vi "Periodic Tasks.vi"() -> ()   [LabVIEW 2011]
doc: "This VI runs in parallel to other tasks. It can contain as many user-defined periodic loops as you need. These can carry out PID or other sorts of timed response."
uses:
  <vilib>/Rock Robotics/SystemInterfaces/Utilities/FPGA_UtilitiesLED State.ctl
  <vilib>/Rock Robotics/SystemInterfaces/Utilities/FPGA_UtilitiesLED Source.ctl
  <vilib>/Rock Robotics/WPI/Relay/WPI_RelayValue.ctl
  Robot Global Data.vi
panel:
  out "Rate":dbl
  out "Heading 2":u16
  out "Angular Rate":dbl
  out "Angle":dbl
  out "Direction":bool
  out "Distance":dbl
  in  "Home Speed":dbl=1.0
  in  "Home Position":dbl=2.85
  out "Current Voltage":dbl
  in  "upper limit":dbl=4.5
  in  "lower limit":dbl=0.85
  # "Speed to move to home"
  # "Target Tracking"
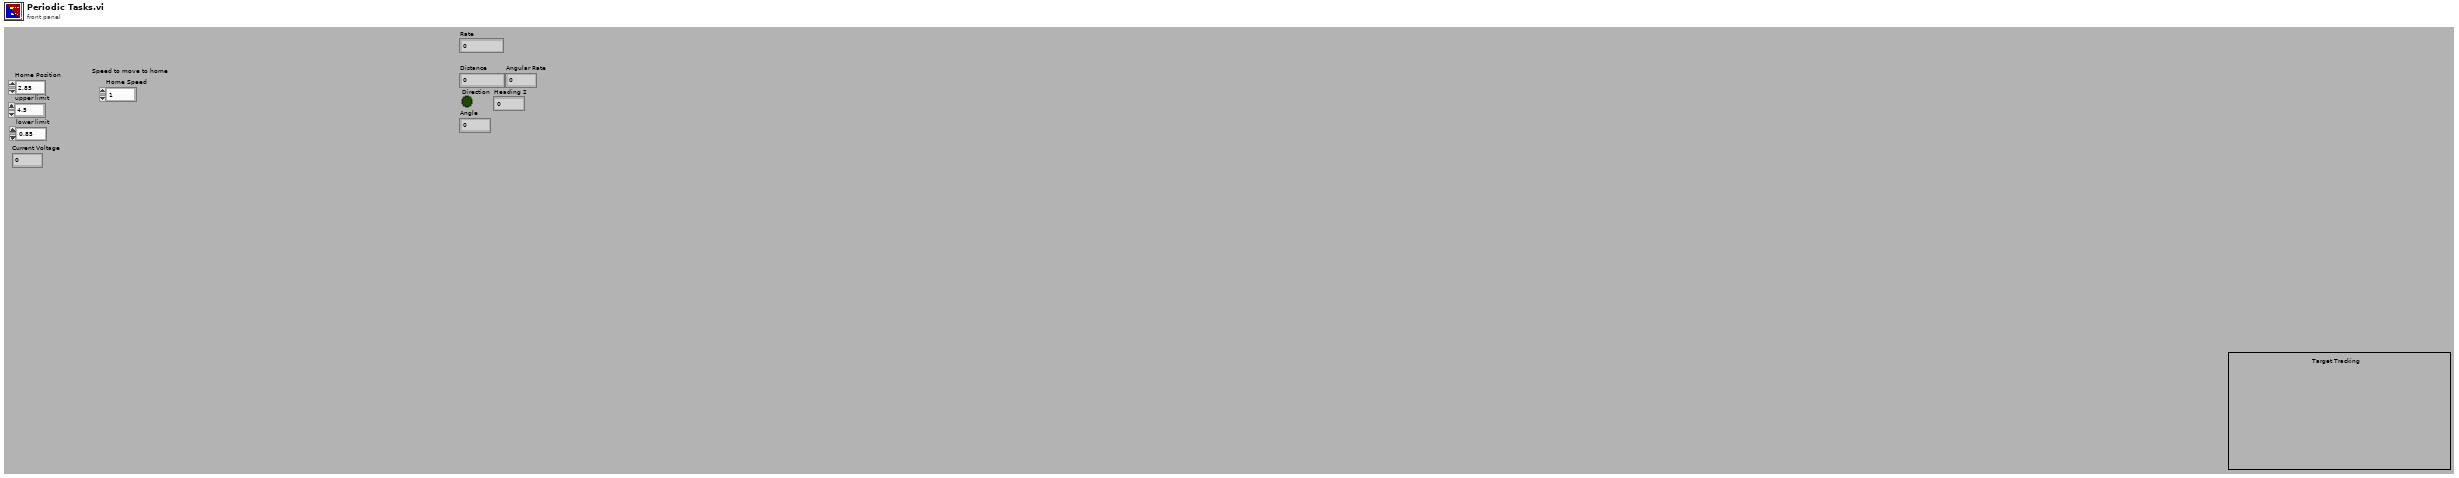
[diagram p1: front panel]
types:
  T1 = typedef "WPI_RelayValue.ctl" = enum16{"Off", "On", "Forward", "Reverse"}
  T2 = typedef "WPI_GyroDevRef.ctl" = cluster{"DevStatus":errorcluster, "Analog Module":T3, "Analog Channel":T4, "Offset":dbl, "Gain (VoltsPerDegree/Second)":dbl}
  T3 = typedef "FPGA_TypedefAnalogModule.ctl" = enum16{"Analog Module 1", "Analog Module 2"}
  T4 = typedef "FPGA_AIChannel.ctl" = enum8{"AI 1", "AI 2", "AI 3", "AI 4", "AI 5", "AI 6", "AI 7", "AI 8", "Invalid"}
  T5 = typedef "WPI_EncoderDevRef.ctl" = cluster{"DevStatus":errorcluster, "EncoderIndex":T6, "CounterIndex":T7, "DistancePerCount":dbl, "Decoding Type":T8}
  T6 = typedef "FPGA_EncoderIdx.ctl" = enum8{"Enc 0", "Enc 1", "Enc 2", "Enc 3", "Invalid"}
  T7 = typedef "FPGA_CounterCtrSystemIndex.ctl" = enum8{"Ctr 0", "Ctr 1", "Ctr 2", "Ctr 3", "Ctr 4", "Ctr 5", "Ctr 6", "Ctr 7", "Invalid"}
  T8 = typedef "WPI_EncoderType.ctl" = enum16{"1x", "2x", "4x"}
  T9 = typedef "WPI_AnalogChannelDevRef.ctl" = cluster{"DevStatus":errorcluster, "Analog Module":T3, "Analog Channel":T4}
  T10 = typedef "WPI_I2CDevRef.ctl" = cluster{"DevStatus":errorcluster, "Digital Module":T11, "Device Address":u8}
  T11 = typedef "FPGA_TypedefDigitalModule.ctl" = enum16{"Digital Module 1", "Digital Module 2"}
  T12 = typedef "WPI_RelayDevRef.ctl" = cluster{"DevStatus":errorcluster, "Relay Channel":T13, "Digital Module":T11, "Relay Direction":T14}
  T13 = typedef "FPGA_DIORelayChannel.ctl" = enum8{"Relay 1", "Relay 2", "Relay 3", "Relay 4", "Relay 5", "Relay 6", "Relay 7", "Relay 8", "Invalid"}
  T14 = typedef "WPI_RelayDirection.ctl" = enum16{"Both directions", "Forward only", "Reverse only"}
  T15 = cluster{"Driver Station Digital Output (1-8)[0]":bool, "Driver Station Digital Output (1-8)[1]":bool, "Driver Station Digital Output (1-8)[2]":bool, "Driver Station Digital Output (1-8)[3]":bool, "Driver Station Digital Output (1-8)[4]":bool, "Driver Station Digital Output (1-8)[5]":bool, "Driver Station Digital Output (1-8)[6]":bool, "Driver Station Digital Output (1-8)[7]":bool, "Driver Station Digital Output (1-8)[8]":bool}
  T16 = typedef "FPGA_UtilitiesLED State.ctl" = enum16{"Off", "On", "Toggle"}
  T17 = typedef "FPGA_UtilitiesLED Source.ctl" = enum16{"User LED", "FPGA LED"}
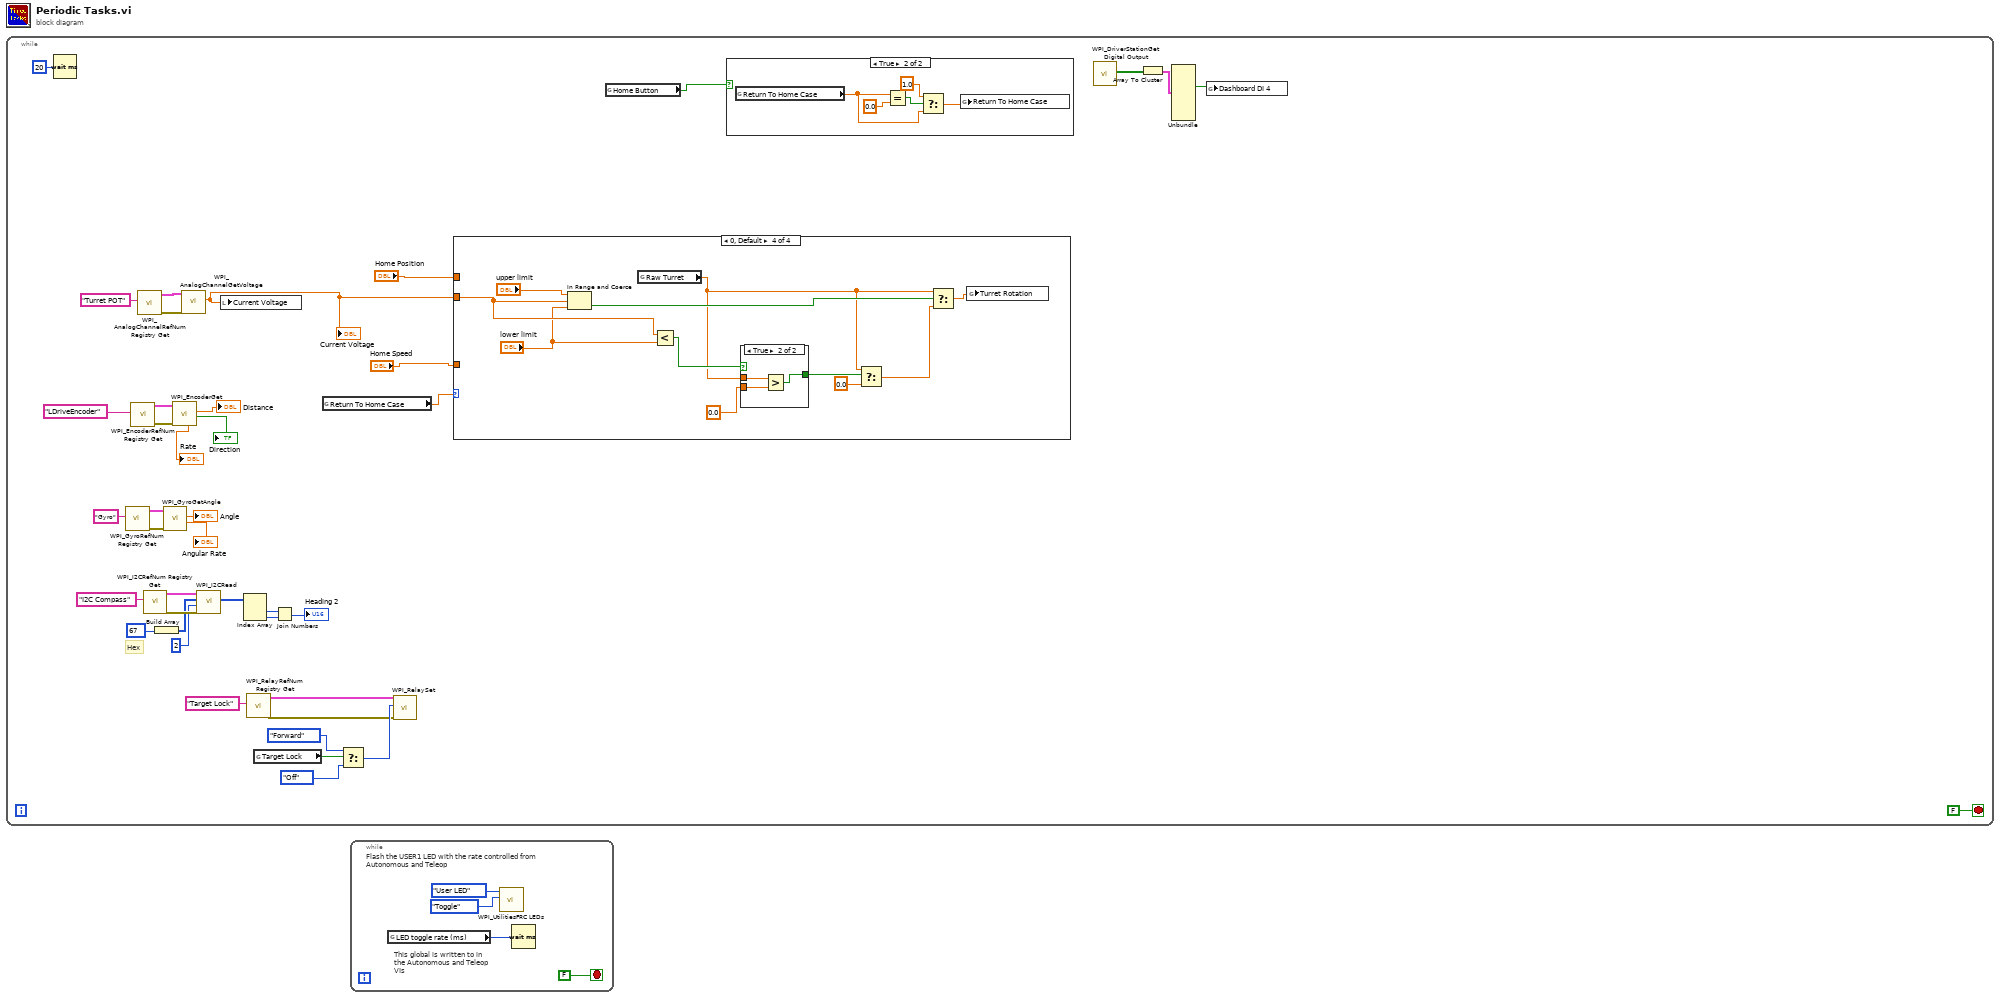
[diagram p0: block diagram]
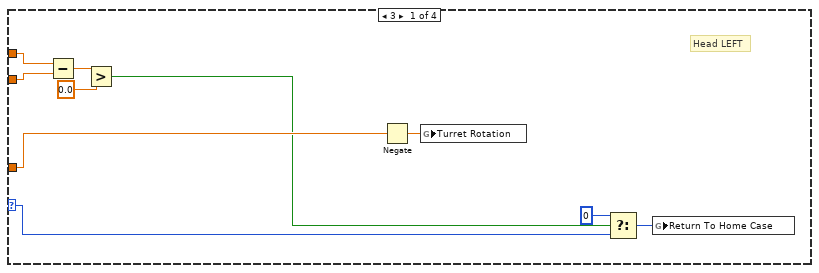
[diagram p2: hidden frame]
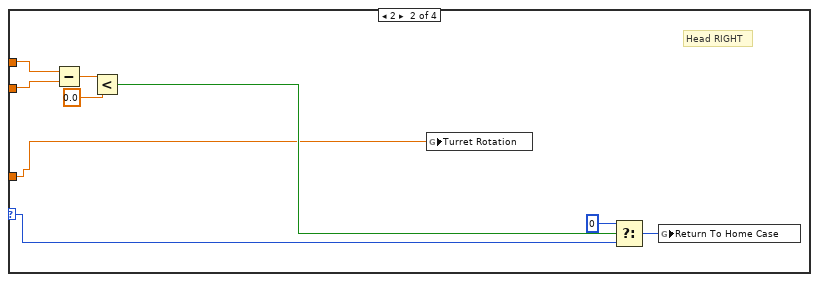
[diagram p3: hidden frame]
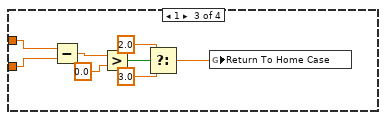
[diagram p4: hidden frame]
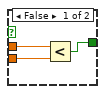
[diagram p5: hidden frame]
diagram:
  n1 = while {
    stop <- FALSE stop-if-true
    # "Hex"
    n2 = Wait (ms)(milliseconds to wait=u32 20) -> ()  [unwired: 1 out]
    n3 = call <vilib>:"WPI_GyroRefNum Registry Get.vi"("refnum name"="Gyro") -> ("error out"=w14:errorcluster, "GyroDevRef"=w15:T2)  [unwired: 9 in]
    n4 = call <vilib>:"WPI_EncoderRefNum Registry Get.vi"("refnum name"="LDriveEncoder") -> ("error out"=w18:errorcluster, "EncoderDevRef"=w19:T5)  [unwired: 9 in]
    n5 = call <vilib>:"WPI_AnalogChannelRefNum Registry Get.vi"("refnum name"="Turret POT") -> ("error out"=w21:errorcluster, "AIDeviceRef"=w22:T9)  [unwired: 9 in]
    n6 = call <vilib>:"WPI_I2CRefNum Registry Get.vi"("refnum name"="I2C Compass") -> ("error out"=w10:errorcluster, "I2CDevRef"=w9:T10)  [unwired: 9 in]
    n7 = Build Array(67) -> (w1:i32[])
    n8 = call <vilib>:"WPI_GyroGetAngle.vi"("error in (no error)"=w14, "GyroDevRef"=w15) -> ("Angular Rate"=→"Angular Rate":dbl, "Angle"=→"Angle":dbl)  [unwired: 6 in, 2 out]
    n9 = call <vilib>:"WPI_EncoderGet.vi"("error in (no error)"=w18, "EncoderDevRef"=w19) -> ("Direction"=→"Direction":bool, "Distance"=→"Distance":dbl, "Rate"=→"Rate":dbl)  [unwired: 4 in, 3 out]
    n10 = call <vilib>:"WPI_AnalogChannelGetVoltage.vi"("error in (no error)"=w21, "AIDeviceRef"=w22) -> ("Voltage"=w30:dbl)  [unwired: 7 in, 2 out]
    "Current Voltage" <- w30
    n11 = call <vilib>:"WPI_I2CRead.vi"("error in (no error)"=w10, "I2CBytesToRead"=u8 2, "I2CRegister"=w1, "I2CDevRef"=w9) -> ("Data Out"=w7:u8[])  [unwired: 5 in, 2 out]
    n12 = local write "Current Voltage"(w30) -> ()
    n13 = Index Array(array=w7) -> (element #1=w5:u8, element #2=w6:u8)  [unwired: 2 in]
    n14 = call <vilib>:"WPI_RelayRefNum Registry Get.vi"("refnum name"="Target Lock") -> ("error out"=w32:errorcluster, "RelayDevRef"=w33:T12)  [unwired: 9 in]
    n15 = global read "Robot Global Data.vi" "Target Lock"() -> (w38:bool)
    n16 = Join Numbers(hi=w5, lo=w6) -> ((hi.lo)=→"Heading 2":u16)
    n17 = global read "Robot Global Data.vi" "Return To Home Case"() -> (w29:dbl)
    n18 = Select(t=WPI_RelayValue."Forward" ("RelayValue"), s=w38, f=WPI_RelayValue."Off" ("RelayValue")) -> (s? t:f=w35:T1)
    n19 = call <vilib>:"WPI_RelaySet.vi"("error in (no error)"=w32, "RelayValue"=w35, "RelayDevRef"=w33) -> ()  [unwired: 7 in, 2 out]
    n20 = case shown="0, Default" w29 {
      selector: w29 -> [w49 w53 _ _]
      tunnel: w30 -> [w45 w54 w67 w79]
      tunnel: "Home Position" -> [w46 w55 w68 _]
      tunnel: "Home Speed" -> [w47 w52 _ _]
      frame 3 {
        # "Head LEFT"
        n21 = Subtract(x=w46, y=w45) -> (x-y=w44:dbl)
        n22 = Greater?(x=w44, y=0.0) -> (0:w42:bool)
        n23 = Negate(x=w47) -> (-x=w48:dbl)
        n24 = global write "Robot Global Data.vi" "Turret Rotation"(w48) -> ()
        n25 = Select(t=0, s=w42, f=w49) -> (s? t:f=w50:i32)
        n26 = global write "Robot Global Data.vi" "Return To Home Case"(w50) -> ()
      }
      frame 2 {
        # "Head RIGHT"
        n27 = Subtract(x=w55, y=w54) -> (x-y=w58:dbl)
        n28 = Less?(x=w58, y=0.0) -> (x < y?=w56:bool)
        n29 = global write "Robot Global Data.vi" "Turret Rotation"(w52) -> ()
        n30 = Select(t=0, s=w56, f=w53) -> (s? t:f=w59:i32)
        n31 = global write "Robot Global Data.vi" "Return To Home Case"(w59) -> ()
      }
      frame 1 {
        n32 = Subtract(x=w68, y=w67) -> (x-y=w66:dbl)
        n33 = Greater?(x=w66, y=0.0) -> (0:w64:bool)
        n34 = Select(t=2.0, s=w64, f=3.0) -> (s? t:f=w61:dbl)
        n35 = global write "Robot Global Data.vi" "Return To Home Case"(w61) -> ()
      }
      frame 0, Default {
        n36 = In Range and Coerce(upper limit="upper limit", x=w79, lower limit="lower limit") -> (In Range?=w76:bool)  [unwired: 1 out]
        n37 = global read "Robot Global Data.vi" "Raw Turret"() -> (w69:dbl)
        n38 = Less?(x=w79, y="lower limit") -> (x < y?=w71:bool)
        n39 = case shown="True" w71 {
          tunnel: 0.0 -> [w81 w85]
          tunnel: [w80 w84] -> w72
          tunnel: w69 -> [w82 w83]
          frame False {
            n40 = Less?(x=w82, y=w81) -> (x < y?=w80:bool)
          }
          frame True {
            n41 = Greater?(x=w83, y=w85) -> (0:w84:bool)
          }
        }
        n42 = Select(t=w69, s=w72, f=0.0) -> (s? t:f=w70:dbl)
        n43 = Select(t=w69, s=w76, f=w70) -> (s? t:f=w78:dbl)
        n44 = global write "Robot Global Data.vi" "Turret Rotation"(w78) -> ()
      }
    }
    n45 = global read "Robot Global Data.vi" "Home Button"() -> (w26:bool)
    n46 = case shown="True" w26 {
      frame False {
      }
      frame True {
        n47 = global read "Robot Global Data.vi" "Return To Home Case"() -> (w87:dbl)
        n48 = Equal?(x=w87, y=0.0) -> (x = y?=w89:bool)
        n49 = Select(t=1.0, s=w89, f=w87) -> (s? t:f=w86:dbl)
        n50 = global write "Robot Global Data.vi" "Return To Home Case"(w86) -> ()
      }
    }
    n51 = call <vilib>:"WPI_DriverStationGet Digital Output.vi"() -> ("Driver Station Digital Output (1-8)"=w41:bool[])  [unwired: 10 in, 1 out]
    n52 = Array To Cluster(array=w41) -> (cluster=w40:T15)
    n53 = Unbundle(w40) -> ("Driver Station Digital Output (1-8)[3]"=w39:bool)  [unwired: 8 out]
    n54 = global write "Robot Global Data.vi" "Dashboard DI 4"(w39) -> ()
  }
  n55 = while {
    stop <- FALSE stop-if-true
    # "This global is written to in the Autonomous and Teleop VIs"
    # "Flash the USER1 LED with the rate controlled from Autonomous and Teleop"
    n56 = global read "Robot Global Data.vi" "LED toggle rate (ms)"() -> (w91:u32)
    n57 = call <vilib>:"WPI_UtilitiesFRC LEDs.vi"("State"=FPGA_UtilitiesLED_State."Toggle", "LED Type"=FPGA_UtilitiesLED_Source."User LED") -> ()  [unwired: 1 in, 9 out]
    n58 = Wait (ms)(milliseconds to wait=w91) -> ()  [unwired: 1 out]
  }
